vi "GOMDBTS2048 spectral Set Enabled.vi"(8 "error in (no error)":errorcluster, 10 "enabled":bool, 11 "handle":i32) -> (0 "error out":errorcluster, 3 "function return":i32)   [LabVIEW 2015, in "GOMDBTS2048.lvlib"]
doc: "GOBTS2048DLL int __stdcall GOMDBTS2048_spectralSetEnabled(int handle, bool enabled);"
uses:
  GOMDBTS2048.lvlib
  runtime/GOMDBTS2048.dll
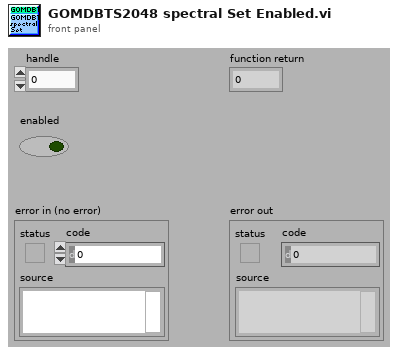
[diagram p1: front panel]
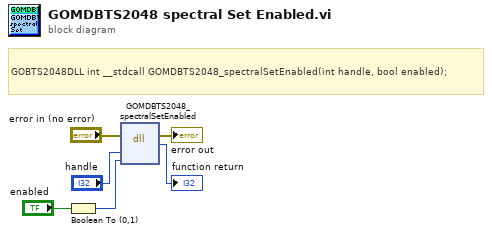
[diagram p0: block diagram]
diagram:
  # "GOBTS2048DLL int __stdcall GOMDBTS2048_spectralSetEnabled(int handle, bool enabled);"
  n1 = Boolean To (0,1)(Boolean="enabled") -> (0, 1=w3:i16)
  n2 = dll-call lib="C:/Users/rkoch/Documents/GO_Library/runtime/GOMDBTS2048.*" fn="GOMDBTS2048_spectralSetEnabled"(error in="error in (no error)", "handle"="handle", "enabled"=w3) -> (error out=→"error out":errorcluster, →"function return":i32)  [unwired: 4 in, 1 out]
